vi "Latch Arcade 2.vi"(11 "Input":bool) -> (3 "Latched":bool)   [LabVIEW 2011]
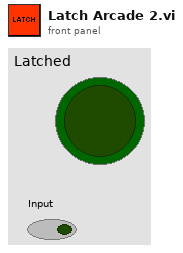
[diagram p1: front panel]
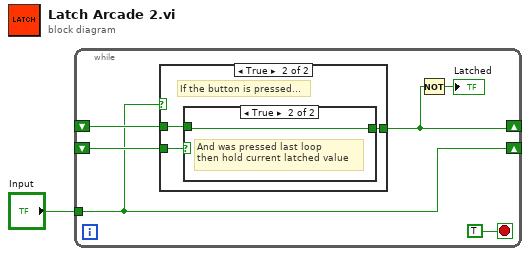
[diagram p0: block diagram]
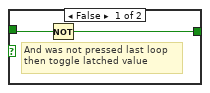
[diagram p3: hidden frame]
diagram:
  n1 = while {
    shift-right: [w3] -> _
    shift-left: _ -> [w7]
    shift-right: [w4] -> _
    shift-left: _ -> [w6]
    tunnel: "Input" -> [w3]
    stop <- TRUE stop-if-true
    n2 = case shown="True" w3 {
      tunnel: w7 -> [_ w11]
      tunnel: w6 -> [w8 w10]
      tunnel: [w8 w9] -> w4
      frame False {
        # "then do nothing"
        # "If button is not pressed"
      }
      frame True {
        # "If the button is pressed..."
        n3 = case shown="True" w11 {
          tunnel: w10 -> [w12 w14]
          tunnel: [w13 w14] -> w9
          frame False {
            # "And was not pressed last loop\nthen toggle latched value"
            n4 = Not(x=w12) -> (.not. x?=w13:bool)
          }
          frame True {
            # "And was pressed last loop\nthen hold current latched value"
          }
        }
      }
    }
    n5 = Not(x=w4) -> (.not. x?=→"Latched":bool)
  }
